vi "Example Kill Program Process.vi"() -> ()   [LabVIEW 2010]
uses:
  C:/tf/play/labview/Tinkerforge.dll
  Tinkerforge.dll
panel:
  out "result":string
  in  "program identifier":string="foobar"
  in  "uid":string="XXYYZZ"
  in  "port":i32=4223
  in  "host":string="localhost"
  # "FIXME: Limited to 63 characters"
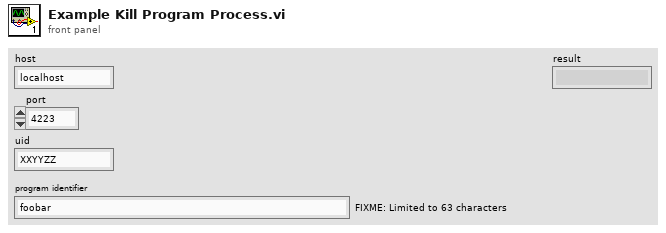
[diagram p1: front panel]
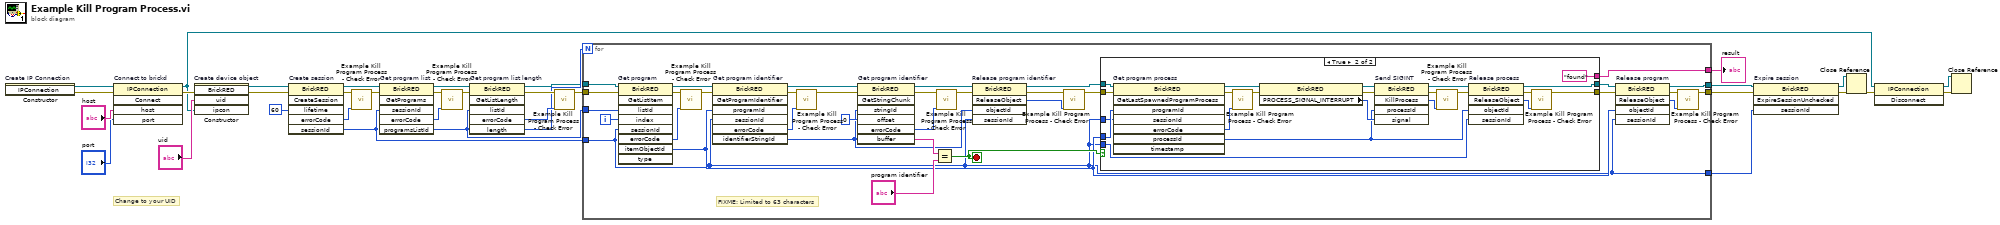
[diagram p0: block diagram]
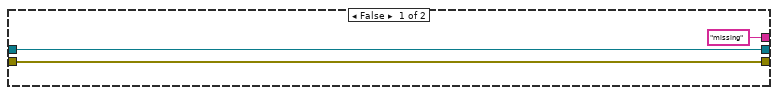
[diagram p2: hidden frame]
diagram:
  # "Change to your UID"
  n1 = constructor on="Create IP Connection" class="IPConnection"() -> (reference out=w34:refnum<k24>, error out=w23:errorcluster)  [unwired: 3 in, 1 out]
  n2 = invoke on="Connect to brickd" class="IPConnection" method="Connect"(reference=w34, error in=w23, "host"="host", "port"="port") -> (reference out=w25:refnum<k24>, error out=w30:errorcluster)  [unwired: 1 in, 3 out]
  n3 = constructor on="Create device object" class="BrickRED"(error in=w30, "uid"="uid", "ipcon"=w25) -> (reference out=w28:refnum<k24>, error out=w29:errorcluster)  [unwired: 2 in, 3 out]
  n4 = invoke on="Create session" class="BrickRED" method="CreateSession"(reference=w28, error in=w29, "lifetime"=i64 60) -> (reference out=w16:refnum<k24>, error out=w21:errorcluster, "errorCode"=w20:u8, "sessionId"=w5:i32)  [unwired: 3 in, 2 out]
  n5 = call "Example Kill Program Process - Check Error.vi"("error code"=w20, "error in"=w21) -> ("error out"=w17:errorcluster)  [unwired: 9 in]
  n6 = invoke on="Get program list" class="BrickRED" method="GetPrograms"(reference=w16, error in=w17, "sessionId"=w5) -> (reference out=w12:refnum<k24>, error out=w15:errorcluster, "errorCode"=w14:u8, "programsListId"=w6:i32)  [unwired: 3 in, 2 out]
  n7 = call "Example Kill Program Process - Check Error.vi"("error code"=w14, "error in"=w15) -> ("error out"=w13:errorcluster)  [unwired: 9 in]
  n8 = invoke on="Get program list length" class="BrickRED" method="GetListLength"(reference=w12, error in=w13, "listId"=w6) -> (reference out=w7:refnum<k24>, error out=w11:errorcluster, "errorCode"=w10:u8, "length"=w9:i32)  [unwired: 3 in, 2 out]
  n9 = call "Example Kill Program Process - Check Error.vi"("error code"=w10, "error in"=w11) -> ("error out"=w8:errorcluster)  [unwired: 9 in]
  n10 = for {
    N: w9 -> [_]
    tunnel: w8 -> [w68]
    tunnel: w7 -> [w67]
    tunnel: w6 -> [w66]
    tunnel: w5 -> [w39]
    tunnel: [w39] -> w4
    tunnel: [w44] -> w3
    tunnel: [w43] -> w2
    tunnel: [w40] -> w1
    i -> [w65]
    stop <- w51 stop-if-true
    # "FIXME: Limited to 63 characters"
    n11 = invoke on="Get program" class="BrickRED" method="GetListItem"(reference=w67, error in=w68, "listId"=w66, "index"=w65, "sessionId"=w39) -> (reference out=w62:refnum<k24>, error out=w64:errorcluster, "errorCode"=w63:u8, "itemObjectId"=w47:i32)  [unwired: 4 in, 5 out]
    n12 = call "Example Kill Program Process - Check Error.vi"("error code"=w63, "error in"=w64) -> ("error out"=w61:errorcluster)  [unwired: 9 in]
    n13 = invoke on="Get program identifier" class="BrickRED" method="GetProgramIdentifier"(reference=w62, error in=w61, "programId"=w47, "sessionId"=w39) -> (reference out=w56:refnum<k24>, error out=w60:errorcluster, "errorCode"=w59:u8, "identifierStringId"=w48:i32)  [unwired: 3 in, 3 out]
    n14 = call "Example Kill Program Process - Check Error.vi"("error code"=w59, "error in"=w60) -> ("error out"=w57:errorcluster)  [unwired: 9 in]
    n15 = invoke on="Get program identifier" class="BrickRED" method="GetStringChunk"(reference=w56, error in=w57, "stringId"=w48, "offset"=i64 0) -> (reference out=w49:refnum<k24>, error out=w55:errorcluster, "errorCode"=w54:u8, "buffer"=w53:string)  [unwired: 3 in, 3 out]
    n16 = Equal?(x=w53, y="program identifier") -> (x = y?=w51:bool)
    n17 = call "Example Kill Program Process - Check Error.vi"("error code"=w54, "error in"=w55) -> ("error out"=w50:errorcluster)  [unwired: 9 in]
    n18 = invoke on="Release program identifier" class="BrickRED" method="ReleaseObject"(reference=w49, error in=w50, "objectId"=w48, "sessionId"=w39) -> (reference out=w35:refnum<k24>, error out=w42:errorcluster, "ReleaseObject"=w41:u8)  [unwired: 1 in, 2 out]
    n19 = call "Example Kill Program Process - Check Error.vi"("error code"=w41, "error in"=w42) -> ("error out"=w36:errorcluster)  [unwired: 9 in]
    n20 = case shown="True" w51 {
      tunnel: w47 -> [_ w93]
      tunnel: ["missing" "found"] -> w40
      tunnel: w39 -> [_ w89]
      tunnel: w39 -> [_ w80]
      tunnel: [w69 w77] -> w38
      tunnel: [w70 w76] -> w37
      tunnel: w36 -> [w69 w73]
      tunnel: w35 -> [w70 w72]
      frame False {
      }
      frame True {
        n21 = invoke on="Get program process" class="BrickRED" method="GetLastSpawnedProgramProcess"(reference=w72, error in=w73, "programId"=w93, "sessionId"=w89) -> (reference out=w83:refnum<k24>, error out=w92:errorcluster, "errorCode"=w90:u8, "processId"=w81:i32)  [unwired: 4 in, 4 out]
        n22 = call "Example Kill Program Process - Check Error.vi"("error code"=w90, "error in"=w92) -> ("error out"=w86:errorcluster)  [unwired: 9 in]
        n23 = property class="BrickRED"(reference=w83, error in=w86) -> (reference out=w84:refnum<k24>, error out=w85:errorcluster, "PROCESS_SIGNAL_INTERRUPT"=w82:u8)
        n24 = invoke on="Send SIGINT" class="BrickRED" method="KillProcess"(reference=w84, error in=w85, "processId"=w81, "signal"=w82) -> (reference out=w78:refnum<k24>, error out=w88:errorcluster, "KillProcess"=w87:u8)  [unwired: 1 in, 2 out]
        n25 = call "Example Kill Program Process - Check Error.vi"("error code"=w87, "error in"=w88) -> ("error out"=w79:errorcluster)  [unwired: 9 in]
        n26 = invoke on="Release process" class="BrickRED" method="ReleaseObject"(reference=w78, error in=w79, "objectId"=w81, "sessionId"=w80) -> (reference out=w76:refnum<k24>, error out=w75:errorcluster, "ReleaseObject"=w74:u8)  [unwired: 1 in, 2 out]
        n27 = call "Example Kill Program Process - Check Error.vi"("error code"=w74, "error in"=w75) -> ("error out"=w77:errorcluster)  [unwired: 9 in]
      }
    }
    n28 = invoke on="Release program" class="BrickRED" method="ReleaseObject"(reference=w37, error in=w38, "objectId"=w47, "sessionId"=w39) -> (reference out=w43:refnum<k24>, error out=w45:errorcluster, "ReleaseObject"=w46:u8)  [unwired: 1 in, 2 out]
    n29 = call "Example Kill Program Process - Check Error.vi"("error code"=w46, "error in"=w45) -> ("error out"=w44:errorcluster)  [unwired: 9 in]
  }
  "result" <- w1
  n30 = invoke on="Expire session" class="BrickRED" method="ExpireSessionUnchecked"(reference=w2, error in=w3, "sessionId"=w4) -> (reference out=w19:refnum<k24>, error out=w18:errorcluster)  [unwired: 1 in, 2 out]
  n31 = Close Reference(reference=w19, error in (no error)=w18) -> (error out=w27:errorcluster)
  n32 = invoke class="IPConnection" method="Disconnect"(reference=w25, error in=w27) -> (reference out=w24:refnum<k24>, error out=w26:errorcluster)  [unwired: 1 in, 1 out]
  n33 = Close Reference(reference=w24, error in (no error)=w26) -> ()  [unwired: 1 out]
